vi "0xED_Read_all_parameters_of_type_int.vi"(8 "error in":errorcluster, 11 "paramUnicorn":T1={"conParam"={"ReadIntParam"=TRUE, "ReadDescrParam"=FALSE, "ReadFloatParam"=TRUE, "debug"=FALSE, "ReadJSON"=TRUE, "IP_address"="192.168.1.216", "N_attempts"=3, "type_con"=enum."TCP", "MB_address"=1, "VISA"="COM1", "connection ID"=refnum, "nameDevices"="", "timeout"=3000, "port"=2000, "type_version"="0F0C0001", "baud_rate"=115200, "VersionControl"=TRUE, "TCP_conn"=TRUE, "WindowSize"=700}, "Param"={"NumParam"={"NTelem"=201, "NInt"=16, "NFloat"=10, "NTable"=2}, "ParamInt"=[{"ID"="Режим работы", "Num"=0, "Name"="", "Type"="", "Enum"="", "Desc"="", "Unit"="", "Access"="", "FormatStr"="", "Min"=0, "Max"=0}, {"ID"="", "Num"=0, "Name"="", "Type"="", "Enum"="", "Desc"="", "Unit"="", "Access"="", "FormatStr"="", "Min"=0, "Max"=0}, {"ID"="", "Num"=0, "Name"="", "Type"="", "Enum"="", "Desc"="", "Unit"="", "Access"="", "FormatStr"="", "Min"=0, "Max"=0}, {"ID"="", "Num"=0, "Name"="", "Type"="", "Enum"="", "Desc"="", "Unit"="", "Access"="", "FormatStr"="", "Min"=0, "Max"=0}, {"ID"="", "Num"=0, "Name"="", "Type"="", "Enum"="", "Desc"="", "Unit"="", "Access"="", "FormatStr"="", "Min"=0, "Max"=0}, {"ID"="", "Num"=0, "Name"="", "Type"="", "Enum"="", "Desc"="", "Unit"="", "Access"="", "FormatStr"="", "Min"=0, "Max"=0}, {"ID"="ModeWork", "Num"=0, "Name"="", "Type"="", "Enum"="", "Desc"="", "Unit"="", "Access"="", "FormatStr"="", "Min"=0, "Max"=0}], "Telemetry"=[], "Table"=[], "ParamFloat"=[]}}) -> (0 "error out":errorcluster, 1 "ArrayIntStr":string[][](array[string]), 2 "ArrayInt":i32[](array[numeric]), 3 "paramUnicorn 2":T1={"conParam"={"ReadIntParam"=TRUE, "ReadDescrParam"=FALSE, "ReadFloatParam"=TRUE, "debug"=FALSE, "ReadJSON"=TRUE, "IP_address"="192.168.1.216", "N_attempts"=3, "type_con"=enum."TCP", "MB_address"=1, "VISA"="COM1", "connection ID"=refnum, "nameDevices"="", "timeout"=3000, "port"=2000, "type_version"="0F0C0001", "baud_rate"=115200, "VersionControl"=TRUE, "TCP_conn"=TRUE, "WindowSize"=700}, "Param"={"NumParam"={"NTelem"=201, "NInt"=16, "NFloat"=10, "NTable"=2}, "ParamInt"=[{"ID"="Режим работы", "Num"=0, "Name"="", "Type"="", "Enum"="", "Desc"="", "Unit"="", "Access"="", "FormatStr"="", "Min"=0, "Max"=0}, {"ID"="", "Num"=0, "Name"="", "Type"="", "Enum"="", "Desc"="", "Unit"="", "Access"="", "FormatStr"="", "Min"=0, "Max"=0}, {"ID"="", "Num"=0, "Name"="", "Type"="", "Enum"="", "Desc"="", "Unit"="", "Access"="", "FormatStr"="", "Min"=0, "Max"=0}, {"ID"="", "Num"=0, "Name"="", "Type"="", "Enum"="", "Desc"="", "Unit"="", "Access"="", "FormatStr"="", "Min"=0, "Max"=0}, {"ID"="", "Num"=0, "Name"="", "Type"="", "Enum"="", "Desc"="", "Unit"="", "Access"="", "FormatStr"="", "Min"=0, "Max"=0}, {"ID"="", "Num"=0, "Name"="", "Type"="", "Enum"="", "Desc"="", "Unit"="", "Access"="", "FormatStr"="", "Min"=0, "Max"=0}, {"ID"="ModeWork", "Num"=0, "Name"="", "Type"="", "Enum"="", "Desc"="", "Unit"="", "Access"="", "FormatStr"="", "Min"=0, "Max"=0}], "Telemetry"=[], "Table"=[], "ParamFloat"=[]}})   [LabVIEW 2017, in "LV_Unicorn.lvlib"]
uses:
  LV_Unicorn.lvlib
  Control/unicorn_Param.ctl
  Control/unicorn_conn.ctl
  Control/unicorn_JSON.ctl
  Control/unicorn_ParamInt.ctl
  Control/unicorn_Telemetry.ctl
  Control/unicorn_Table.ctl
  Control/unicorn_ParamFloat.ctl
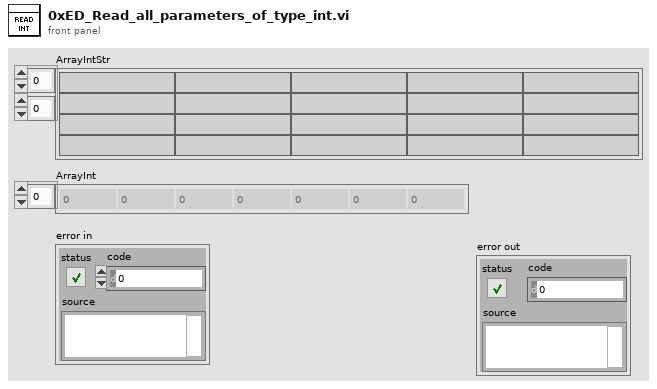
[diagram p1: front panel]
types:
  T1 = typedef "LV_Unicorn.lvlib/unicorn_Param.ctl" = cluster{"conParam":T2, "Param":T3}
  T2 = typedef "LV_Unicorn.lvlib/unicorn_conn.ctl" = cluster{"ReadIntParam":bool, "ReadDescrParam":bool, "ReadFloatParam":bool, "debug":bool, "ReadJSON":bool, "IP_address":string, "N_attempts":i32, "type_con":enum16{"Serial", "TCP"}, "MB_address":i32, "VISA":refnum<visa-resource-name>, "connection ID":refnum<k5>, "nameDevices":string, "timeout":i32, "port":u16, "type_version":string, "baud_rate":u32, "VersionControl":bool, "TCP_conn":bool, "WindowSize":i32}
  T3 = typedef "LV_Unicorn.lvlib/unicorn_JSON.ctl" = cluster{"NumParam":cluster{"NTelem":i32, "NInt":i32, "NFloat":i32, "NTable":i32}, "ParamInt":T4, "Telemetry":T5, "Table":T6, "ParamFloat":T7}
  T4 = typedef "LV_Unicorn.lvlib/unicorn_ParamInt.ctl" = cluster{"ID":string, "Num":i32, "Name":string, "Type":string, "Enum":string, "Desc":string, "Unit":string, "Access":string, "FormatStr":string, "Min":i32, "Max":i32}[]
  T5 = typedef "LV_Unicorn.lvlib/unicorn_Telemetry.ctl" = cluster{"ID":string, "Num":i32, "Name":string, "Desc":string, "Unit":string, "FormatStr":string, "Min":i32, "Max":i32}[]
  T6 = typedef "LV_Unicorn.lvlib/unicorn_Table.ctl" = cluster{"Num":i32, "Access":string, "ColumnCount":i32, "NeedParamPrepare":bool, "Columns":cluster{"Column":i32, "Desc":string, "Name":string}[], "DataType":string, "FormatStr":string, "ID":string, "Name":string, "RowCount":i32, "Rows":cluster{"Desc":string, "ID":string, "Max":i32, "Min":i32, "Name":string, "Row":i32, "Unit":string}[], "Type":string}[]
  T7 = typedef "LV_Unicorn.lvlib/unicorn_ParamFloat.ctl" = cluster{"ID":string, "Num":i32, "Name":string, "Type":string, "Enum":string, "Desc":string, "Unit":string, "Access":string, "FormatStr":string, "Min":sgl, "Max":sgl}[]
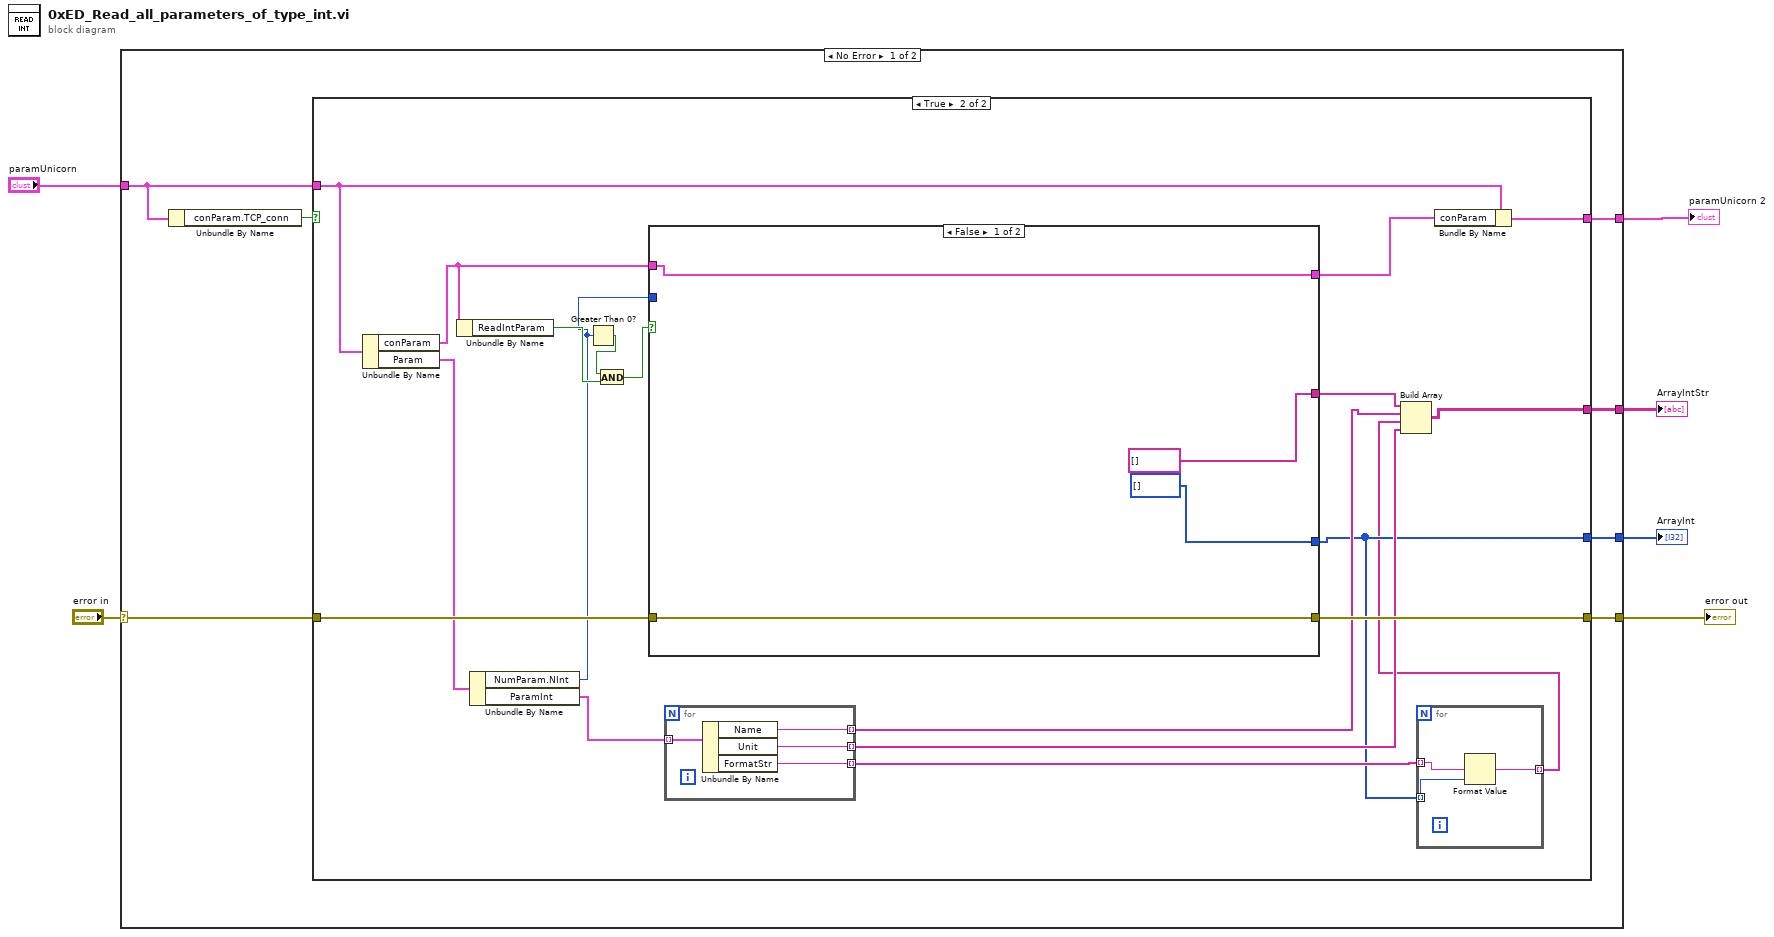
[diagram p0: block diagram]
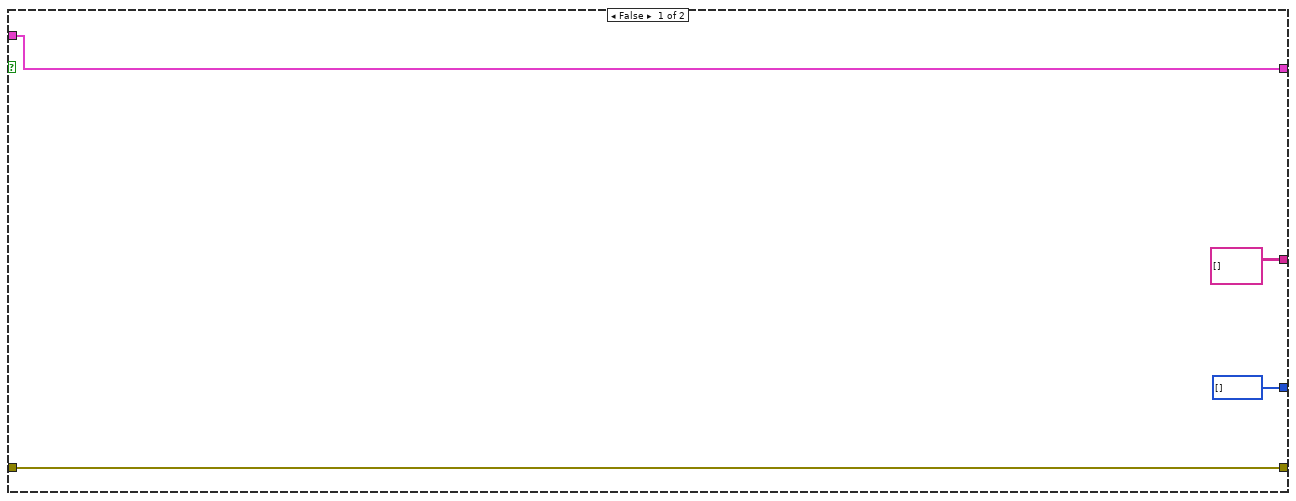
[diagram p2: hidden frame]
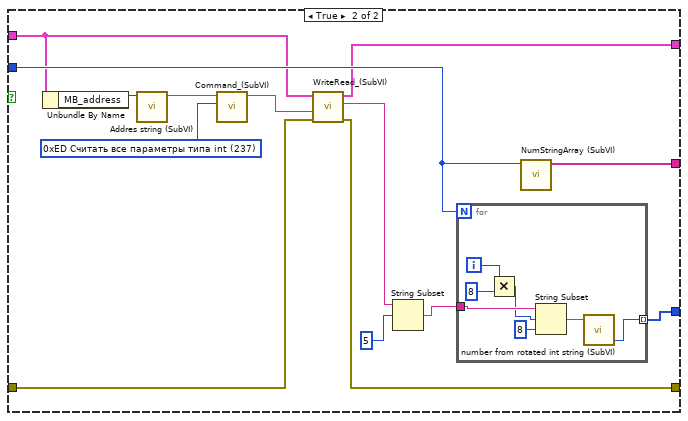
[diagram p3: hidden frame]
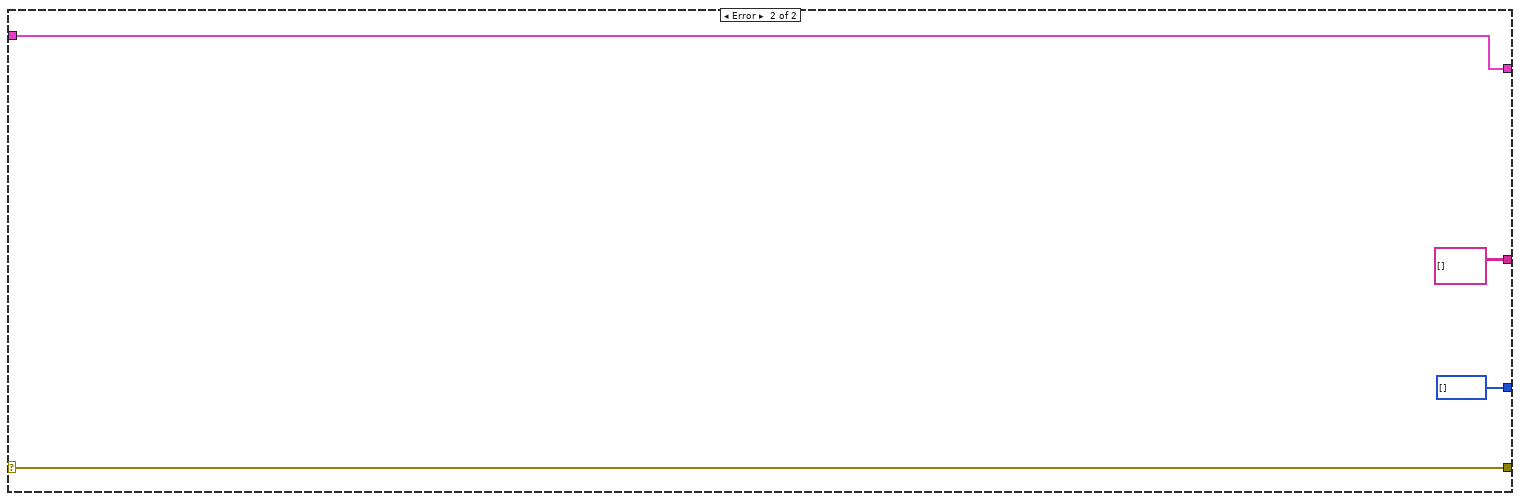
[diagram p4: hidden frame]
diagram:
  n1 = case shown="No Error" "error in" {
    selector: "error in" -> [w12 w72]
    tunnel: [w13 w72] -> w6
    tunnel: "paramUnicorn" -> [w8 w71]
    tunnel: [w11 w71] -> w3
    tunnel: [w10 i32[] []] -> w2
    tunnel: [w9 string[][] []] -> w1
    frame No Error {
      n2 = Unbundle By Name(w8) -> ("conParam.TCP_conn"=w7:bool)
      n3 = case shown="True" w7 {
        tunnel: [w14 w36] -> w13
        tunnel: w12 -> [w14 w34]
        tunnel: w8 -> [w17 w27]
        tunnel: [w17 w25] -> w11
        tunnel: [i32[] [] w19] -> w10
        tunnel: [string[][] [] w24] -> w9
        frame False {
        }
        frame True {
          n4 = Unbundle By Name(w27) -> ("conParam"=w29:T2, "Param"=w28:T3)
          n5 = Unbundle By Name(w29) -> ("ReadIntParam"=w32:bool)
          n6 = Unbundle By Name(w28) -> ("NumParam.NInt"=w30:i32, "ParamInt"=w23:T4)
          n7 = Greater Than 0?(x=w30) -> (x > 0?=w33:bool)
          n8 = And(x=w33, y=w32) -> (x .and. y?=w31:bool)
          n9 = case shown="False" w31 {
            tunnel: [i32[] [] w52] -> w19
            tunnel: [string[] [] ("Array") w58] -> w35
            tunnel: w30 -> [_ w57]
            tunnel: w29 -> [w44 w56]
            tunnel: w34 -> [w46 w54]
            tunnel: [w46 w53] -> w36
            tunnel: [w44 w48] -> w26
            frame False {
            }
            frame True {
              w51 = u16 237 items=["0xE0 Запрос количества доступных параметров"=224, "0xE1 Записать один параметр типа float"=225, "0xE2 Записать один параметр типа int"=226, "0xE3 Считать один параметр телеметрии"=227, "0xE4 Записать все параметры типа float"=228, "0xE5 Записать все параметры типа int"=229, "0xE6 Считать все данные телеметрии"=230, "0xE7 Получить описание одного параметра типа float"=231, "0xE8 Получить описание одного параметра типа int"=232, "0xE9 Получить описание одного параметра телеметрии"=233, "0xEA Считать один параметр типа float"=234, "0xEB Считать один параметр типа int"=235, "0xEC Считать все параметры типа float"=236, "0xED Считать все параметры типа int"=237, "0xEE Считать считать фрагмент описания устройства в формате JSON"=238, "0x06 Записать UUID"=6, "0x07 Чтение UUID"=7, "0x45 Считывание параметров Flash памяти"=69, "0x43 Запись страницы Flash памяти"=67, "0x44 Чтения страницы Flash памяти"=68, "0x46 Получить описание Flash-памяти"=70, "0xFA Программный сброс"=250, "0xFB Изменение скорости интерфейса"=251, "0xFF Считывание типа и версии устройства"=255, "0x50 Запрос кол-ва табличных параметров"=80, "0x51 Запрос описания табличного параметра"=81, "0x52 Чтение данных табличного параметра"=82, "0x53 Запись данных табличного параметра"=83, "0x54 Подготовка табличного параметра"=84, "0x55 Запрос прогресса подготовки табличного параметра"=85, "0x56 Освобождение данных подготовленного табличного параметра"=86] ("Команда")
              n10 = Unbundle By Name(w56) -> ("MB_address"=w55:i32)
              n11 = call "Addres string (SubVI).vi"("Адрес"=w55) -> ("String"=w50:string)  [unwired: 10 in]
              n12 = call "Command_(SubVI).vi"("Команда"=w51, "String in"=w50) -> ("String out"=w49:string)  [unwired: 9 in]
              n13 = call "WriteRead_(SubVI).vi"("error in"=w54, "Запрос"=w49, "ParamIn"=w56) -> ("error out"=w53:errorcluster, "Ответ"=w59:string, "ParamOut"=w48:T2)  [unwired: 4 in, 2 out]
              n14 = String Subset(string=w59, offset (0)=5) -> (substring=w60:string)  [unwired: 1 in]
              n15 = for {
                N: w57 -> [_]
                tunnel: w60 -> [w68]
                tunnel: [w62] -> w52 mode=indexing
                i -> [w65]
                n16 = Multiply(x=w65, y=i8 8) -> (x*y=w64:i32)
                n17 = String Subset(string=w68, offset (0)=w64, length (rest)=8 ("length (rest)")) -> (substring=w63:string)
                n18 = call "number from rotated int string (SubVI).vi"("String"=w63) -> ("int number"=w62:i32)  [unwired: 2 in, 2 out]
              }
              n19 = call "NumStringArray (SubVI).vi"("NInt"=w57) -> ("Array"=w58:string[])  [unwired: 10 in]
            }
          }
          n20 = for {
            tunnel: w23 -> [w43] mode=indexing
            tunnel: [w42] -> w22 mode=indexing
            tunnel: [w41] -> w21 mode=indexing
            tunnel: [w40] -> w20 mode=indexing
            n21 = Unbundle By Name(w43) -> ("Name"=w42:string, "Unit"=w41:string, "FormatStr"=w40:string)
          }
          n22 = for {
            tunnel: w20 -> [w39] mode=indexing
            tunnel: w19 -> [w38] mode=indexing
            tunnel: [w37] -> w18 mode=indexing
            n23 = Format Value(format string=w39, value (0)=w38) -> (output string=w37:string)  [unwired: 1 in]
          }
          n24 = Build Array(w35, w22, w18, w21) -> (w24:string[][])
          n25 = Bundle By Name(cluster=w27, "conParam"=w26) -> (w25:T1)
        }
      }
    }
    frame Error {
    }
  }
  "error out" <- w6
  "paramUnicorn 2" <- w3
  "ArrayInt" <- w2
  "ArrayIntStr" <- w1
